vi "Traverse_Space.vi"(9 "Show Panel?":bool, 10 "Traverse Setup":string) -> (3 "Error Comments":string)   [LabVIEW 2015]
doc: "This is an example of using features of the VI Server as a client. It shows how you might browse from one or more applications that may be exporting data from one or more data stations. \n\nThe example shows how to query a server for its list of exported VIs, how to get references to the VIs, and how call them with the Call By Reference function."
uses:
  Route mapping/Exclude_cluster.ctl
  Route mapping/Box_size.ctl
  Route mapping/Exclusion_type.ctl
  Controls/ok_button.ctl
  Globals/Constants_global.vi
  Route mapping/Route_mapping_global.vi
  Globals/Trav_pos_global.vi
panel:
  in  "Probe Support":T1=[{"Max"=15.0, "Min"=-15.0}, {"Max"=250.0, "Min"=0.0}, {"Max"=15.0, "Min"=-15.0}] {"Min" format="%#.1f"; "Max" format="%#.1f"}
  in  "Traverse space filename":u16(ring) items=["Default_Space_file.xls", "heelo.xls", "hello_test1.xls", "---Save As---"]
  in  "Traverse Name":u16(ring) items=["A_Tunnel", "Aero_Enclosure", "Aero_Sting", "Aero_ThroughWall", "Aero_Tunnel", "Angle_Calibrator", "B_Tunnel", "D_Tunnel", "dummy", "Dummy_Traverse", "EnFlo_", "EnFlo_Measure_Height", "EnFlo_Stack", "EnFlo_Stack  dfg", "EnFlo_Trav3", "EnFlo_Trav4", "EnFlo_Tunnel", "EnFlo_Turntable", "F1_Wing_Angle", "Fruit_Rig", "Hello_5.xls", "Laser_Disp_Scanner", "Laser_Meas_Traverse", "None", "Pitch_Traverse", "Pitch_Yaw", "PIV_Traverse", "Pressure_Port_1", "Pressure_Port_2", "Scanning Valve", "Soil_Rig", "Tank"]
  out "Message":string
  in  "Cancel Button":bool
  in  "OK":T2
  in  "Traverse Limits":T1=[{"Max"=15001.0, "Min"=12000.0}, {"Max"=1000.0, "Min"=-1000.0}, {"Max"=700.0, "Min"=0.0}] {"Min" format="%#.1f"; "Max" format="%#.1f"}
  in  "Probe Volume":T1=[{"Max"=15.0, "Min"=-15.0}, {"Max"=250.0, "Min"=0.0}, {"Max"=15.0, "Min"=-15.0}] {"Min" format="%#.1f"; "Max" format="%#.1f"}
  in  "Exclude Array":T3[](array[typedef])=[{"Sizes"=[{"Max"=15000.0, "Min"=0.0}, {"Max"=1000.0, "Min"=-1000.0}, {"Max"=300.0, "Min"=0.0}], "Name"="Roughness Elements", "Exclude Type"=enum."Allow only vertical moves"}, {"Sizes"=[{"Max"=17000.0, "Min"=16000.0}, {"Max"=200.0, "Min"=-200.0}, {"Max"=-50.0, "Min"=-250.0}], "Name"="B204", "Exclude Type"=enum."Exclude completely"}] {"Sizes"."Min" format="%#.1f"; "Sizes"."Max" format="%#.1f"}
  # "Enter all coordinates assuming the Model Orientation is zero degrees"
  # "(Relative to measurement position)"
  # "X                           Y                          Z"
  # "X                           Y                          Z"
  # "(Relative to measurement position)"
  # "(Relative to measurement position)"
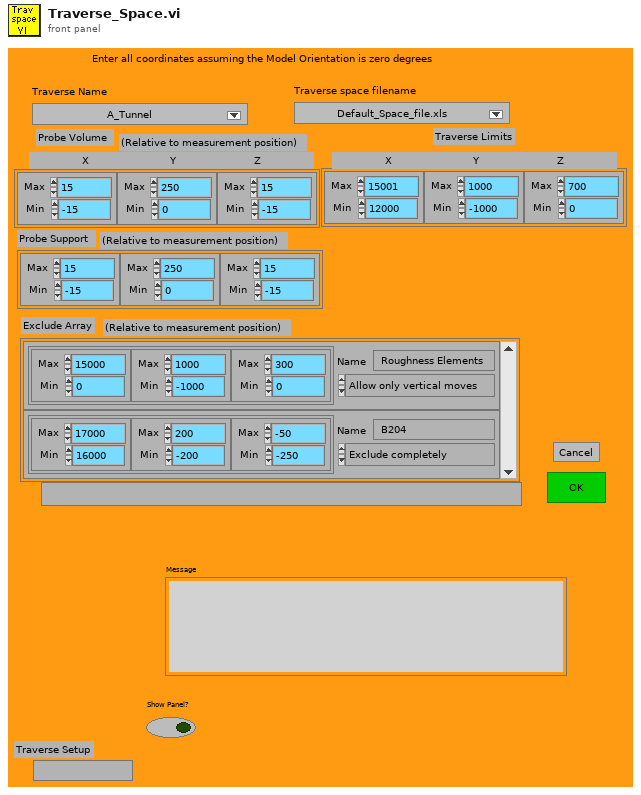
[diagram p1: front panel]
types:
  T1 = typedef "Box_size.ctl" = cluster{"Max":sgl, "Min":sgl}[]
  T2 = typedef "ok_button.ctl" = bool
  T3 = typedef "Exclude_cluster.ctl" = cluster{"Sizes":T1, "Name":string, "Exclude Type":T4}
  T4 = typedef "Exclusion_type.ctl" = enum16{"Exclude completely", "Allow only vertical moves"}
  T5 = enum16{"Load setup from excel file", "Save setup to excel file"}
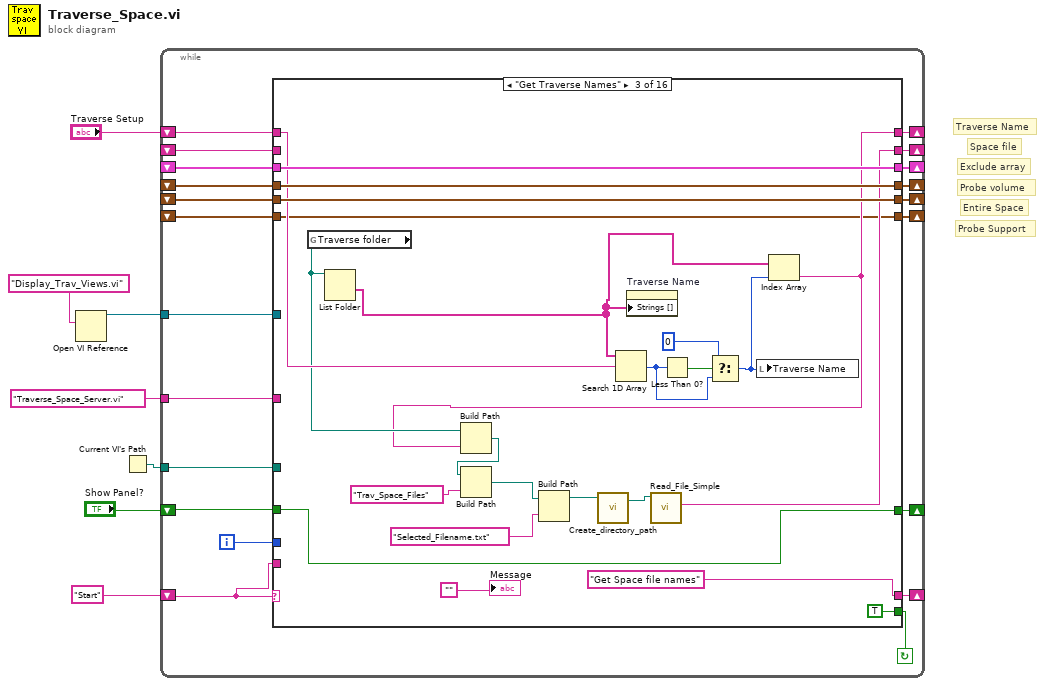
[diagram p0: block diagram]
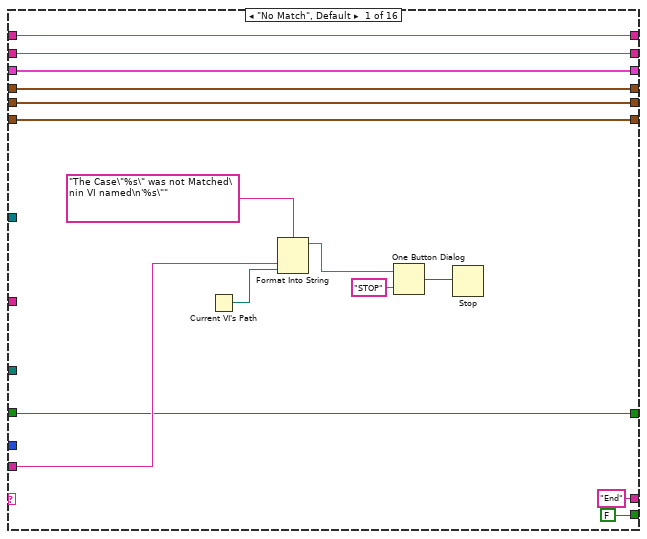
[diagram p2: hidden frame]
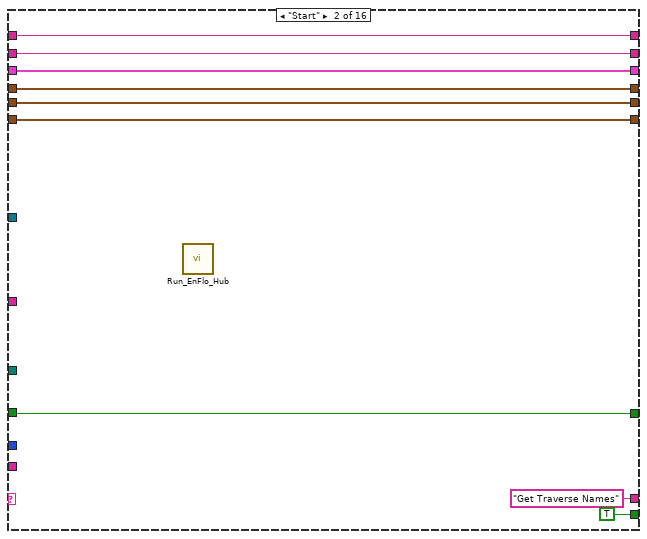
[diagram p3: hidden frame]
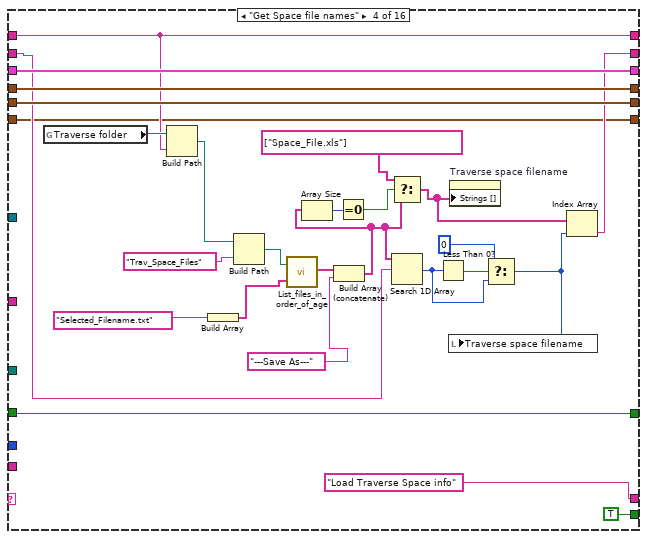
[diagram p4: hidden frame]
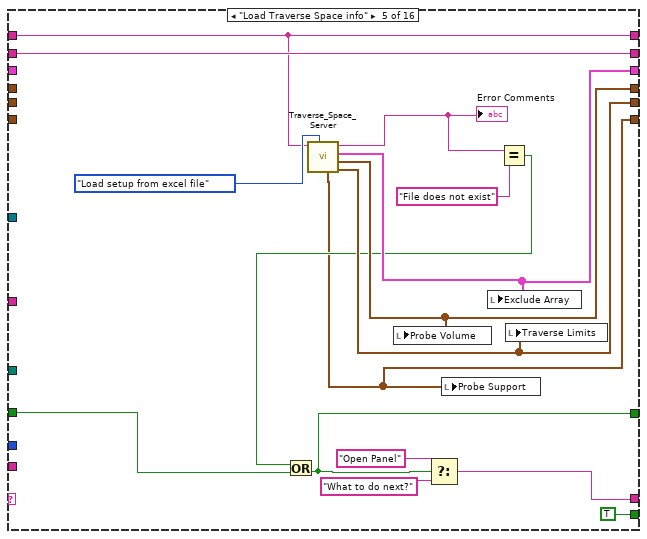
[diagram p5: hidden frame]
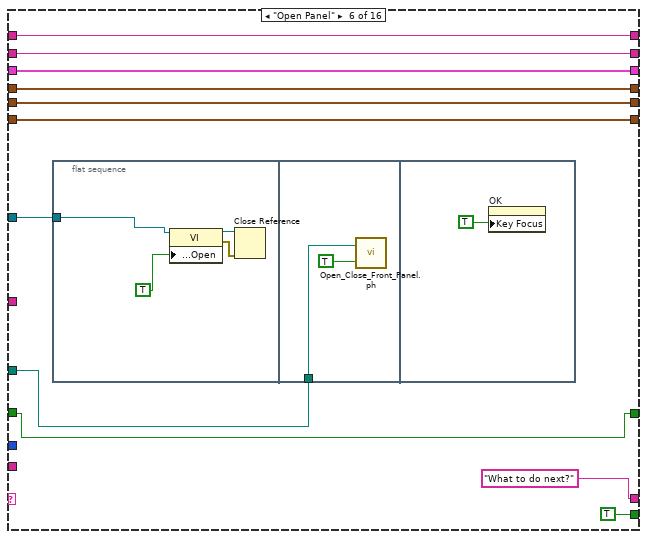
[diagram p6: hidden frame]
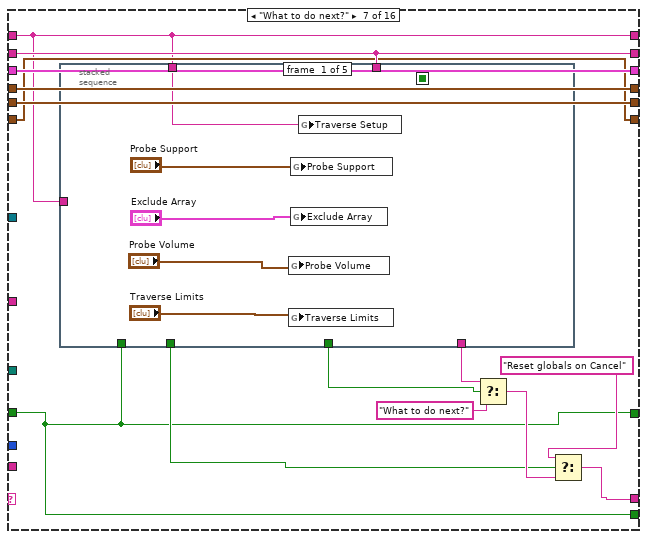
[diagram p7: hidden frame]
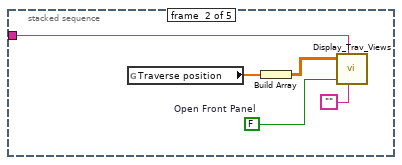
[diagram p8: hidden frame]
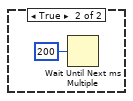
[diagram p10: hidden frame]
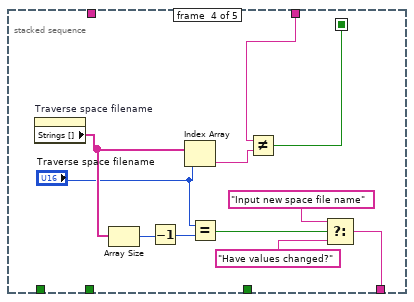
[diagram p11: hidden frame]
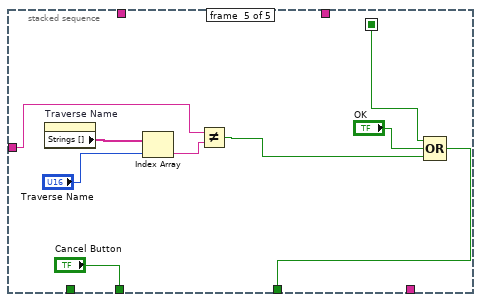
[diagram p12: hidden frame]
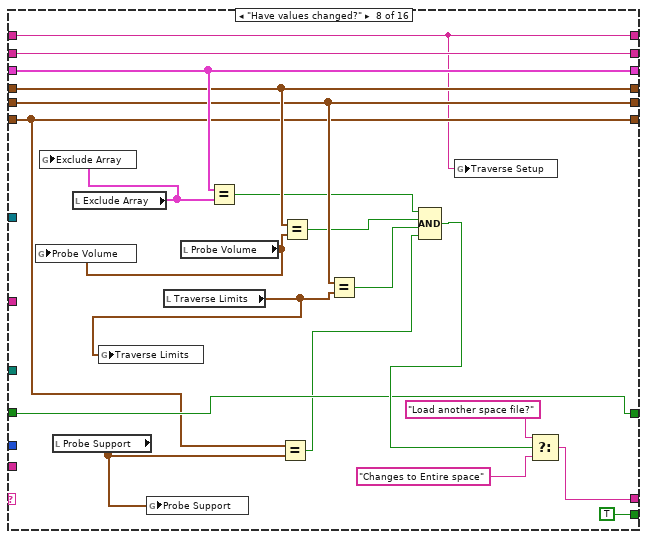
[diagram p13: hidden frame]
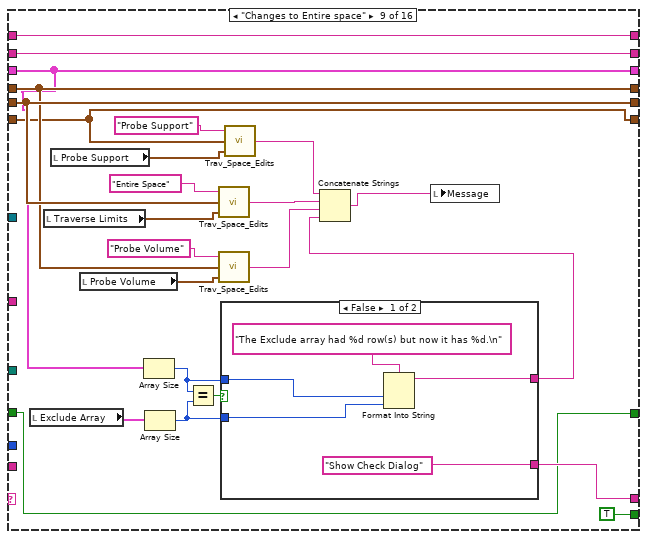
[diagram p14: hidden frame]
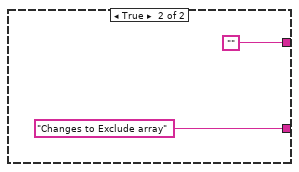
[diagram p15: hidden frame]
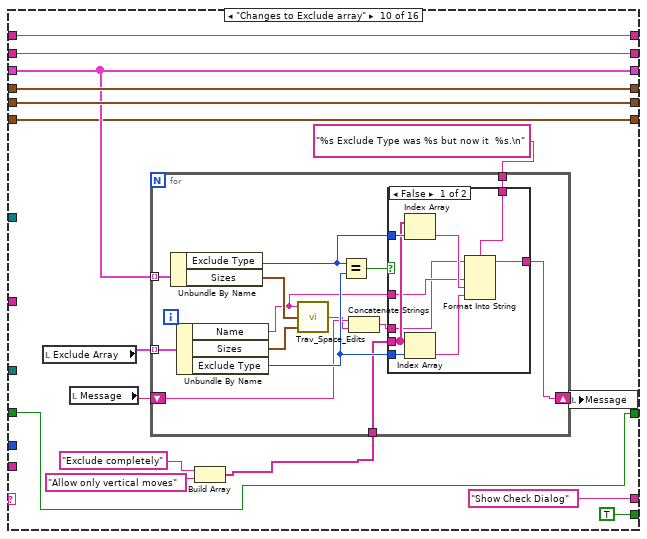
[diagram p16: hidden frame]
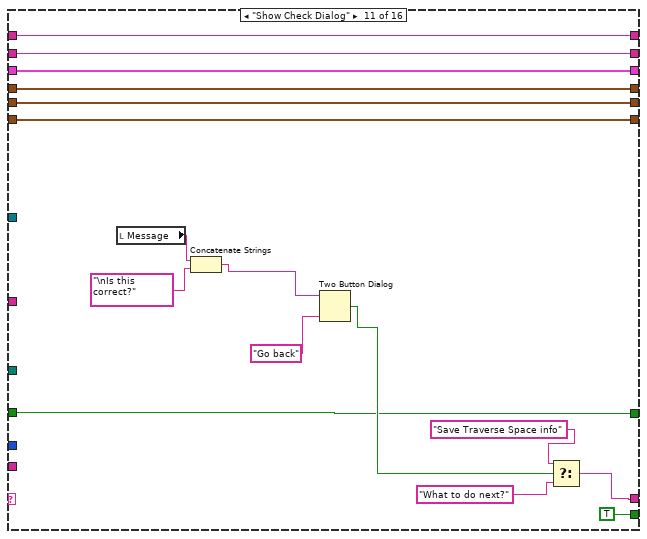
[diagram p18: hidden frame]
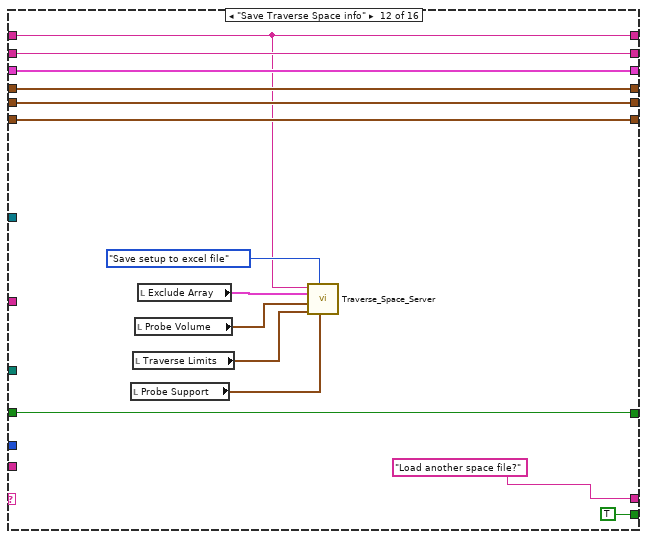
[diagram p19: hidden frame]
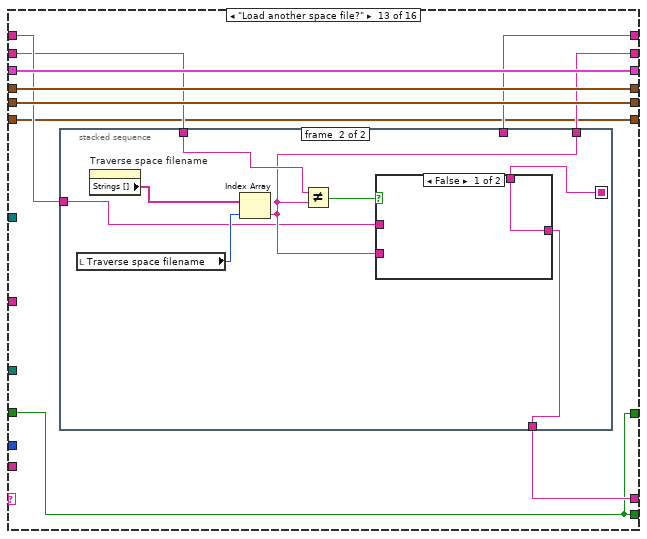
[diagram p20: hidden frame]
diagram:
  # "Probe Support"
  # "Traverse Name"
  # "Space file"
  # "Entire Space"
  # "Probe volume"
  # "Exclude array"
  n1 = Open VI Reference(vi path="Display_Trav_Views.vi") -> (vi reference=w1:refnum<vi>)  [unwired: 1 in, 5 out]
  n2 = Current VI's Path() -> (path=w5:path)
  n3 = while {
    tunnel: "Traverse_Space_Server.vi" ("VI name to run on server") -> [w26]
    shift-left: "Start" -> [w23]
    shift-right: [w25] -> _
    tunnel: w5 -> [w24]
    shift-right: [w22] -> _
    shift-left: _ -> [w19]
    shift-right: [w21] -> _
    shift-left: _ -> [w18]
    shift-right: [w20] -> _
    shift-left: _ -> [w17]
    shift-right: [w15] -> _
    shift-left: "Traverse Setup" -> [w13]
    shift-right: [w16] -> _
    shift-left: _ -> [w14]
    shift-right: [w11] -> _
    shift-left: "Show Panel?" -> [w12]
    tunnel: w1 -> [w10]
    shift-right: [w9] -> _
    shift-left: _ -> [w8]
    i -> [w28]
    stop <- w27 continue-if-true
    n4 = case shown="\"Get Traverse Names\"" w23 {
      tunnel: w28 -> [_ _ _ _ _ _ _ _ _ _ _ _ _ _ _ _]
      tunnel: [FALSE ("status") TRUE ("status") TRUE ("status") TRUE ("status") TRUE ("status") TRUE ("status") w137 TRUE ("status") TRUE ("status") TRUE ("status") TRUE ("status") TRUE ("status") w305 w337 TRUE ("status") FALSE ("status")] -> w27
      tunnel: ["End" ("f") "Get Traverse Names" ("f") "Get Space file names" "Load Traverse Space info" w117 "What to do next?" w149 w192 w215 "Show Check Dialog" ("f") w279 "Load another space file?" w306 w338 "Close Panel" "End"] -> w25
      tunnel: w26 -> [_ _ _ _ _ _ _ _ _ _ _ _ _ _ _ _]
      tunnel: w12 -> [w30 w45 w54 w77 w107 w121 w137 w190 w208 w235 w275 w293 w305 w337 w362 w374]
      tunnel: w24 -> [_ _ _ _ _ w124 _ _ _ _ _ _ _ _ _ w388]
      tunnel: w23 -> [w38 _ _ _ _ _ _ _ _ _ _ _ _ _ _ _]
      tunnel: [w35 w52 w73 w100 w116 w127 w147 w202 w218 w245 w289 w301 w313 w346 w367 w387] -> w22
      tunnel: [w34 w51 w72 w99 w115 w126 w146 w201 w220 w247 w288 w300 w312 w345 w366 w386] -> w21
      tunnel: [w33 w50 w71 w98 w114 w125 w145 w200 w224 w248 w286 w299 w311 w344 w365 w385] -> w20
      tunnel: w19 -> [w35 w52 w73 w100 _ w127 w147 w202 w218 w245 w289 w301 w313 w346 w367 w387]
      tunnel: w18 -> [w34 w51 w72 w99 _ w126 w146 w201 w220 w247 w288 w300 w312 w345 w366 w386]
      tunnel: w17 -> [w33 w50 w71 w98 _ w125 w145 w200 w224 w248 w286 w299 w311 w344 w365 w385]
      tunnel: [w31 w46 w56 w83 w110 w122 w142 w191 w209 w236 w276 w294 w307 w340 w363 w375] -> w16
      tunnel: [w32 w47 w62 w82 w103 w123 w138 w183 w210 w237 w277 w290 w309 w334 w360 w380] -> w15
      tunnel: w14 -> [w31 w46 _ w81 w110 w122 w142 w191 w209 w236 w276 w294 w308 w335 w363 w375]
      tunnel: w13 -> [w32 w47 w65 w82 w103 w123 w138 w183 w210 w237 w277 w290 w310 w334 w360 w380]
      tunnel: [w30 w45 w54 w77 w105 w121 w137 w190 w208 w235 w275 w293 w305 w337 w362 w374] -> w11
      tunnel: w10 -> [_ _ _ _ _ w120 _ _ _ _ _ _ _ _ _ w370]
      tunnel: [w29 w44 w53 w76 w104 w119 w139 w185 w203 w234 w274 w292 w304 w336 w361 w369] -> w9
      tunnel: w8 -> [w29 w44 w53 w76 _ w119 w139 w185 w203 w234 w274 w292 w304 w336 w361 w369]
      frame "No Match", Default {
        n5 = Current VI's Path() -> (path=w43:path)
        n6 = Format Into String(format string="The Case\"%s\" was not Matched\nin VI named\n'%s\"" ("Format String"), w38, w43) -> (resulting string=w40:string)  [unwired: 2 in, 1 out]
        n7 = One Button Dialog(message=w40, button name ("OK")="STOP") -> (true=w42:bool)
        n8 = Stop(stop? (T)=w42) -> ()
      }
      frame "Start" {
        n9 = call "Run_EnFlo_Hub.vi"() -> ()  [unwired: 8 out]
      }
      frame "Get Traverse Names" {
        n10 = global read "Constants_global.vi" "Traverse folder"() -> (w63:path)
        n11 = List Folder(path=w63) -> (folder names=w55:string[])  [unwired: 1 in, 5 out]
        n12 = Search 1D Array(1D array=w55, element=w65) -> (index of element=w68:i32)  [unwired: 1 out]
        n13 = property on="Traverse Name" class="Ring (strict)"("Strings []"=w55) -> ()  [unwired: 2 in, 2 out]
        n14 = Less Than 0?(x=w68) -> (x < 0?=w69:bool)
        n15 = Select(t=0, s=w69, f=w68) -> (s? t:f=w66:i32)
        n16 = local write "Traverse Name"(w66) -> ()
        n17 = Index Array(array=w55, index=w66) -> (element=w62:string)
        n18 = Build Path(base path=w63, name or relative path=w62) -> (appended path=w61:path)
        n19 = Build Path(base path=w61, name or relative path="Trav_Space_Files" ("Substring")) -> (appended path=w60:path)
        n20 = Build Path(base path=w60, name or relative path="Selected_Filename.txt" ("Substring")) -> (appended path=w57:path)
        n21 = call "Create_directory_path.vi"("Path name"=w57) -> ("Path name Out"=w58:path)  [unwired: 2 in, 1 out]
        n22 = call "Read_File_Simple.vi"("Filename"=w58) -> ("string"=w56:string)  [unwired: 2 in, 7 out]
        "Message" <- ""
      }
      frame "Get Space file names" {
        n23 = global read "Constants_global.vi" "Traverse folder"() -> (w94:path)
        n24 = Build Path(base path=w94, name or relative path=w82) -> (appended path=w92:path)
        n25 = Build Array("Selected_Filename.txt" ("Substring")) -> (w91:string[])
        n26 = Build Path(base path=w92, name or relative path="Trav_Space_Files" ("Substring")) -> (appended path=w84:path)
        n27 = call "List_files_in_order_of_age.vi"("Files to Hide"=w91, "Folder"=w84) -> ("file names"=w80:string[])
        n28 = Build Array (concatenate)(w80, "---Save As---") -> (w79:string[])
        n29 = Array Size(array=w79) -> (size(s)=w89:i32)
        n30 = Equal To 0?(x=w89) -> (x = 0?=w88:bool)
        n31 = Select(t=string[] ["Space_File.xls"] ("appended array"), s=w88, f=w79) -> (s? t:f=w86:string[])
        n32 = Search 1D Array(1D array=w79, element=w81) -> (index of element=w96:i32)  [unwired: 1 out]
        n33 = Less Than 0?(x=w96) -> (x < 0?=w97:bool)
        n34 = property on="Traverse space filename" class="Ring (strict)"("Strings []"=w86) -> ()  [unwired: 2 in, 2 out]
        n35 = Select(t=0, s=w97, f=w96) -> (s? t:f=w85:i32)
        n36 = local write "Traverse space filename"(w85) -> ()
        n37 = Index Array(array=w86, index=w85) -> (element=w83:string)
      }
      frame "Load Traverse Space info" {
        n38 = call "Traverse_Space_Server.vi"("Mode"=T5."Load setup from excel file", "Traverse Name"=w103) -> ("Traverse Limits Out"=w114:T1, "Probe Volume Out"=w115:T1, "Exclude Array Out"=w116:T3[], "Error Comments"=w108:string, "Probe Support Out"=w104:T1)  [unwired: 4 in, 1 out]
        "Error Comments" <- w108
        n39 = local write "Probe Volume"(w115) -> ()
        n40 = local write "Probe Support"(w104) -> ()
        n41 = local write "Exclude Array"(w116) -> ()
        n42 = Equal?(x=w108, y="File does not exist") -> (x = y?=w106:bool)
        n43 = Or(x=w106, y=w107) -> (x .or. y?=w105:bool)
        n44 = Select(t="Open Panel", s=w105, f="What to do next?") -> (s? t:f=w117:string)
        n45 = local write "Traverse Limits"(w114) -> ()
      }
      frame "Open Panel" {
        n46 = flat-sequence {
          tunnel: w120 -> [w130]
          tunnel: w124 -> [w134]
          frame #0 {
            n47 = property class="VI"(reference=w130, "Front Panel Window:Open"=TRUE) -> (reference out=w132:refnum<vi>, error out=w131:errorcluster)  [unwired: 1 in]
            n48 = Close Reference(reference=w132, error in (no error)=w131) -> ()  [unwired: 1 out]
          }
          frame #1 {
            n49 = call "Open_Close_Front_Panel.ph.vi"("Front Panel Window:Open"=TRUE, "VI path"=w134) -> ()  [unwired: 2 out]
          }
          frame #2 {
            n50 = property on="OK" class="Bool"("Key Focus"=TRUE) -> ()  [unwired: 2 in, 2 out]
          }
        }
      }
      frame "What to do next?" {
        n51 = stacked-sequence {
          seq-local: [_ _ _ w167 _] -> [_ _ _ _ w174]
          tunnel: w138 -> [_ w156 _ _ w179]
          tunnel: [_ _ _ _ w175] -> w144
          tunnel: [_ _ _ _ "Cancel Button"] -> w143
          tunnel: w142 -> [_ _ _ w168 _]
          tunnel: [_ _ _ w164 _] -> w140
          tunnel: w138 -> [w151 _ _ _ _]
          tunnel: w137 -> [_ _ w161 _ _]
          frame #0 {
            n52 = global write "Route_mapping_global.vi" "Probe Volume"("Probe Volume") -> ()
            n53 = global write "Route_mapping_global.vi" "Traverse Limits"("Traverse Limits") -> ()
            n54 = global write "Route_mapping_global.vi" "Probe Support"("Probe Support") -> ()
            n55 = global write "Route_mapping_global.vi" "Exclude Array"("Exclude Array") -> ()
            n56 = global write "Route_mapping_global.vi" "Traverse Setup"(w151) -> ()
          }
          frame #1 {
            w157 = FALSE  # Open Front Panel
            n57 = global read "Trav_pos_global.vi" "Traverse position"() -> (w158:sgl[])
            n58 = Build Array(w158) -> (w159:sgl[][])
            n59 = call "Display_Trav_Views.vi"("Current Probe Position"=w159, "Traverse Name"=w156, "Open Front Panel"=w157, "Error Comments"="") -> ()  [unwired: 3 in, 4 out]
          }
          frame #2 {
            n60 = case shown="False" w161 {
              frame False {
              }
              frame True {
                n61 = Wait Until Next ms Multiple(millisecond multiple=u32 200) -> ()  [unwired: 1 out]
              }
            }
          }
          frame #3 {
            n62 = property on="Traverse space filename" class="Ring (strict)"() -> ("Strings []"=w170:string[])  [unwired: 2 in, 2 out]
            n63 = Array Size(array=w170) -> (size(s)=w172:i32)
            n64 = Decrement(x=w172) -> (x-1=w171:i32)
            n65 = Index Array(array=w170, index="Traverse space filename") -> (element=w173:string)
            n66 = Equal?(x="Traverse space filename", y=w171) -> (x = y?=w166:bool)
            n67 = Not Equal?(x=w168, y=w173) -> (x != y?=w167:bool)
            n68 = Select(t="Input new space file name" ("f"), s=w166, f="Have values changed?") -> (s? t:f=w164:string)
          }
          frame #4 {
            n69 = property on="Traverse Name" class="Ring (strict)"() -> ("Strings []"=w180:string[])  [unwired: 2 in, 2 out]
            n70 = Index Array(array=w180, index="Traverse Name") -> (element=w178:string)
            n71 = Not Equal?(x=w179, y=w178) -> (x != y?=w177:bool)
            n72 = Compound Arithmetic op=OR(w174, "OK", w177) -> (w175:T2)
          }
        }
        n73 = Select(t=w140, s=w144, f="What to do next?") -> (s? t:f=w150:string)
        n74 = Select(t="Reset globals on Cancel", s=w143, f=w150) -> (s? t:f=w149:string)
      }
      frame "Have values changed?" {
        n75 = local read "Probe Support"() -> (w186:T1)
        n76 = local read "Exclude Array"() -> (w189:T3[])
        n77 = global write "Route_mapping_global.vi" "Exclude Array"(w189) -> ()
        n78 = global write "Route_mapping_global.vi" "Probe Support"(w186) -> ()
        n79 = local read "Traverse Limits"() -> (w187:T1)
        n80 = global write "Route_mapping_global.vi" "Traverse Limits"(w187) -> ()
        n81 = local read "Probe Volume"() -> (w188:T1)
        n82 = global write "Route_mapping_global.vi" "Probe Volume"(w188) -> ()
        n83 = Equal?(x=w202, y=w189) -> (x = y?=w199:bool)
        n84 = Equal?(x=w185, y=w186) -> (x = y?=w184:bool)
        n85 = Equal?(x=w201, y=w188) -> (x = y?=w198:bool)
        n86 = Equal?(x=w200, y=w187) -> (x = y?=w197:bool)
        n87 = Compound Arithmetic op=AND(w199, w198, w197, w184) -> (w195:bool)
        n88 = global write "Route_mapping_global.vi" "Traverse Setup"(w183) -> ()
        n89 = Select(t="Load another space file?", s=w195, f="Changes to Entire space") -> (s? t:f=w192:string)
      }
      frame "Changes to Entire space" {
        n90 = local read "Exclude Array"() -> (w217:T3[])
        n91 = local read "Traverse Limits"() -> (w223:T1)
        n92 = local read "Probe Support"() -> (w207:T1)
        n93 = local read "Probe Volume"() -> (w221:T1)
        n94 = Array Size(array=w218) -> (size(s)=w214:i32)
        n95 = Array Size(array=w217) -> (size(s)=w213:i32)
        n96 = Equal?(x=w214, y=w213) -> (x = y?=w216:bool)
        n97 = call "Trav_Space_Edits.vi"("New"=w223, "Original"=w224, "Row Name"="Entire Space") -> ("Changes"=w205:string)
        n98 = call "Trav_Space_Edits.vi"("New"=w221, "Original"=w220, "Row Name"="Probe Volume") -> ("Changes"=w219:string)
        n99 = case shown="False" w216 {
          tunnel: ["Show Check Dialog" ("f") "Changes to Exclude array" ("f")] -> w215
          tunnel: w214 -> [w230 _]
          tunnel: w213 -> [w229 _]
          tunnel: [w227 ""] -> w212
          frame False {
            n100 = Format Into String(format string="The Exclude array had %d row(s) but now it has %d.\n", w230, w229) -> (resulting string=w227:string)  [unwired: 2 in, 1 out]
          }
          frame True {
          }
        }
        n101 = call "Trav_Space_Edits.vi"("New"=w207, "Original"=w203, "Row Name"="Probe Support") -> ("Changes"=w204:string)
        n102 = Concatenate Strings(w204, w205, w219, w212) -> (w211:string)
        n103 = local write "Message"(w211) -> ()
      }
      frame "Changes to Exclude array" {
        n104 = local read "Exclude Array"() -> (w246:T3[])
        n105 = local read "Message"() -> (w239:string)
        n106 = Build Array("Exclude completely", "Allow only vertical moves") -> (w242:string[])
        n107 = for {
          tunnel: w245 -> [w261] mode=indexing
          tunnel: w246 -> [w263] mode=indexing
          shift-right: [w253] -> w240
          shift-left: w239 -> [w251]
          tunnel: w242 -> [w256]
          tunnel: "%s Exclude Type was %s but now it  %s.\n" ("format string") -> [w255]
          n108 = Unbundle By Name(w261) -> ("Exclude Type"=w257:T4, "Sizes"=w260:T1)
          n109 = Unbundle By Name(w263) -> ("Name"=w254:string, "Sizes"=w262:T1, "Exclude Type"=w258:T4)
          n110 = call "Trav_Space_Edits.vi"("New"=w262, "Original"=w260, "Row Name"=w254) -> ("Changes"=w250:string)
          n111 = Equal?(x=w257, y=w258) -> (x = y?=w259:bool)
          n112 = Concatenate Strings(w251, w250) -> (w252:string)
          n113 = case shown="False" w259 {
            tunnel: w258 -> [w272 _]
            tunnel: w257 -> [w271 _]
            tunnel: w256 -> [w270 _]
            tunnel: w255 -> [w267 _]
            tunnel: w254 -> [w266 _]
            tunnel: w252 -> [w265 w273]
            tunnel: [w264 w273] -> w253
            frame False {
              n114 = Index Array(array=w270, index=w271) -> (element=w268:string)
              n115 = Index Array(array=w270, index=w272) -> (element=w269:string)
              n116 = Format Into String(format string=w267, initial string=w265, w266, w268, w269) -> (resulting string=w264:string)  [unwired: 1 in, 1 out]
            }
            frame True {
            }
          }
        }
        n117 = local write "Message"(w240) -> ()
      }
      frame "Show Check Dialog" {
        n118 = local read "Message"() -> (w285:string)
        n119 = Concatenate Strings(w285, "\nIs this correct?") -> (w284:string)
        n120 = Two Button Dialog(message=w284, 1:"Go back" ("F button name (\"Cancel\")")) -> (T button?=w281:bool)  [unwired: 1 out]
        n121 = Select(t="Save Traverse Space info", s=w281, f="What to do next?") -> (s? t:f=w279:string)
      }
      frame "Save Traverse Space info" {
        n122 = local read "Probe Support"() -> (w291:T1)
        n123 = local read "Traverse Limits"() -> (w295:T1)
        n124 = local read "Probe Volume"() -> (w296:T1)
        n125 = local read "Exclude Array"() -> (w297:T3[])
        n126 = call "Traverse_Space_Server.vi"("Probe Support"=w291, "Mode"=T5."Save setup to excel file", "Traverse Limits"=w295, "Probe Volume"=w296, "Exclude Array"=w297, "Traverse Name"=w290) -> ()  [unwired: 6 out]
      }
      frame "Load another space file?" {
        n127 = stacked-sequence {
          seq-local: [w315 _] -> [_ w324]
          tunnel: w310 -> [w320 w322]
          tunnel: [w316 _] -> w309
          tunnel: [_ w327] -> w306
          tunnel: w308 -> [_ w326]
          tunnel: [_ w323] -> w307
          frame #0 {
            n128 = local read "Traverse Name"() -> (w314:u16)
            n129 = property on="Traverse Name" class="Ring (strict)"() -> ("Strings []"=w321:string[])  [unwired: 2 in, 2 out]
            n130 = Index Array(array=w321, index=w314) -> (element=w316:string)
            n131 = Not Equal?(x=w320, y=w316) -> (x != y?=w319:bool)
            n132 = Select(t="Get Traverse Names" ("f"), s=w319, f="Close Panel") -> (s? t:f=w315:string)
          }
          frame #1 {
            n133 = local read "Traverse space filename"() -> (w328:u16)
            n134 = property on="Traverse space filename" class="Ring (strict)"() -> ("Strings []"=w329:string[])  [unwired: 2 in, 2 out]
            n135 = Index Array(array=w329, index=w328) -> (element=w323:string)
            n136 = Not Equal?(x=w326, y=w323) -> (x != y?=w325:bool)
            n137 = case shown="False" w325 {
              tunnel: [w330 "Load Traverse Space info" ("f")] -> w327
              tunnel: w324 -> [w330 _]
              tunnel: w323 -> [_ w332]
              tunnel: w322 -> [_ w331]
              frame False {
              }
              frame True {
                n138 = call "Update_Selected_Space_File.vi"("Selected Space File Name"=w332, "Traverse Setup"=w331) -> ()  [unwired: 1 in]
              }
            }
          }
        }
      }
      frame "Input new space file name" {
        n139 = property on="Traverse space filename" class="Ring (strict)"() -> ("Strings []"=w339:string[])  [unwired: 2 in, 2 out]
        n140 = call "Input_String_Dialog.vi"("Message to user"="Please Enter a new  space file name") -> ("Ok Out"=w341:bool, "Output string"=w342:string)  [unwired: 1 in]
        n141 = case shown="True" w341 {
          tunnel: w342 -> [_ w355]
          tunnel: [w348 w350] -> w340
          tunnel: w335 -> [w348 _]
          tunnel: w339 -> [_ w351]
          tunnel: ["What to do next?" ("f") "Save Traverse Space info" ("f")] -> w338
          tunnel: w334 -> [_ w349]
          frame False {
          }
          frame True {
            n142 = call "Fast_string_Replace.vi"("Replace match with:"="_", "Input String"=w355, "regular expression"=" ") -> ("Output String"=w356:string)  [unwired: 2 out]
            n143 = local write "Traverse space filename"(0) -> ()
            n144 = call "Add_filename_suffix.vi"("Filename"=w356, "Suffix to add"=".xls") -> ("Filename out"=w350:string)  [unwired: 3 out]
            n145 = Build Array (concatenate)(w350, w351) -> (w354:string[])
            n146 = property on="Traverse space filename" class="Ring (strict)"("Strings []"=w354) -> ()  [unwired: 2 in, 2 out]
            n147 = call "Update_Selected_Space_File.vi"("Selected Space File Name"=w350, "Traverse Setup"=w349) -> ()  [unwired: 1 in]
          }
        }
      }
      frame "Reset globals on Cancel" {
        n148 = global write "Route_mapping_global.vi" "Traverse Limits"(w365) -> ()
        n149 = global write "Route_mapping_global.vi" "Probe Volume"(w366) -> ()
        n150 = global write "Route_mapping_global.vi" "Exclude Array"(w367) -> ()
        n151 = global write "Route_mapping_global.vi" "Traverse Setup"(w360) -> ()
        n152 = global write "Route_mapping_global.vi" "Probe Support"(w361) -> ()
      }
      frame "Close Panel" {
        w378 = FALSE  # append to file? (new file:F)
        w379 = FALSE  # advisory dialog? (display:T)
        n153 = global read "Constants_global.vi" "Traverse folder"() -> (w384:path)
        n154 = call "Open_Close_Front_Panel.ph.vi"("Front Panel Window:Open"=FALSE, "VI path"=w388) -> ()  [unwired: 2 out]
        n155 = Build Path(base path=w384, name or relative path=w380) -> (appended path=w382:path)
        n156 = Build Path(base path=w382, name or relative path="Trav_Space_Files" ("Substring")) -> (appended path=w381:path)
        n157 = Build Path(base path=w381, name or relative path="Selected_Filename.txt" ("Substring")) -> (appended path=w376:path)
        n158 = property class="VI"(reference=w370, "Front Panel Window:Open"=FALSE) -> (reference out=w372:refnum<vi>, error out=w371:errorcluster)  [unwired: 1 in]
        n159 = Close Reference(reference=w372, error in (no error)=w371) -> ()  [unwired: 1 out]
        n160 = call "Write_Characters_To_File.vi"("file path (dialog if empty)"=w376, "advisory dialog? (display:T)"=w379, "character string"=w375, "append to file? (new file:F)"=w378) -> ()  [unwired: 1 in, 4 out]
      }
    }
  }
